vi "Get SMO Public API.vi"(8 "error in (no error)":errorcluster, 11 "instrument.Cryostation in":refnum<class "instrument.Cryostation.lvclass">) -> (0 "error out":errorcluster, 2 "Commands":string[](array[string]), 3 "instrument.Cryostation out":refnum<class "instrument.Cryostation.lvclass">)   [LabVIEW 2019, in "instrument.Cryostation.lvclass"]
uses:
  instrument.Cryostation.lvclass
  Typedefs/Cryostation.Commands--enum.ctl
  <userlib>/LevyLab/Instrument Framework/Instrument Types/Cryostat/Instrument.Cryostat.lvclass
  <userlib>/LevyLab/Instrument Framework/SMOs/Instrument/Instrument.lvclass
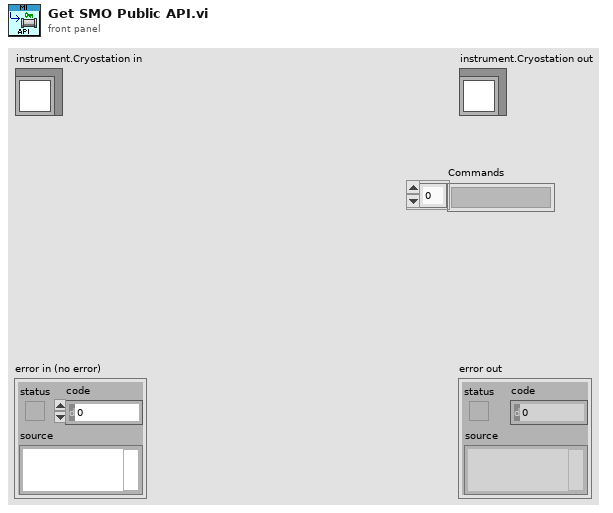
[diagram p1: front panel]
types:
  T1 = typedef "instrument.Cryostation.lvclass/Cryostation.Commands--enum.ctl" = enum16{"Get Temperature"}
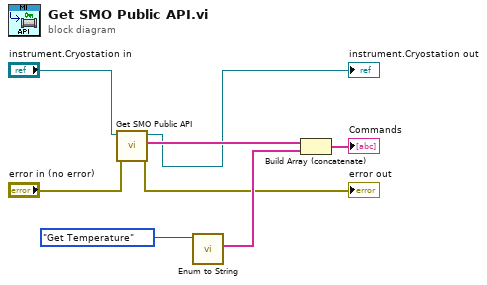
[diagram p0: block diagram]
diagram:
  n1 = call-parent "Get SMO Public API.vi"("error in (no error)"="error in (no error)", "Instrument in"="instrument.Cryostation in") -> ("error out"=→"error out":errorcluster, "Commands"=w6:string[], "Instrument out"=→"instrument.Cryostation out":refnum<class "instrument.Cryostation.lvclass">)  [unwired: 7 in]
  n2 = call <userlib>:"Enum to String.vi"("Command"=Cryostation.Commands--enum."Get Temperature" ("Commands")) -> ("Commands []"=w3:string[])  [unwired: 9 in, 1 out]
  n3 = Build Array (concatenate)(w6, w3) -> (→"Commands":string[])
